vi "Output Powers Saving.vi"(7 "connection information":path, 8 "EFCVoltage":string, 9 "OutputPower":string="40000057.37", 10 "DC_SN":string, 11 "Temperature":string) -> ()   [LabVIEW 2024]
uses:
  <vilib>/addons/database/NI_Database_API.lvlib
  <vilib>/addons/database/_DB Variant To Data/Database Variant To Data.xnode
  <vilib>/addons/database/Connection.llb/DB Tools Open Connec (Path).vi
  <vilib>/addons/database/Connection.llb/Conn Execute.vi
  <vilib>/addons/database/Recordset.llb/Rec Destroy - Connection.vi
panel:
  out "Time Measured":string
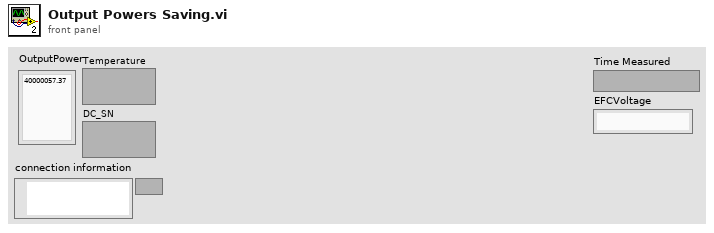
[diagram p1: front panel]
types:
  T1 = typedef "NI_Database_API.lvlib/Conn ObjectReference.ctl" = refnum<k1>
  T2 = typedef "NI_Database_API.lvlib/Rec ObjectReference.ctl" = refnum<k1>
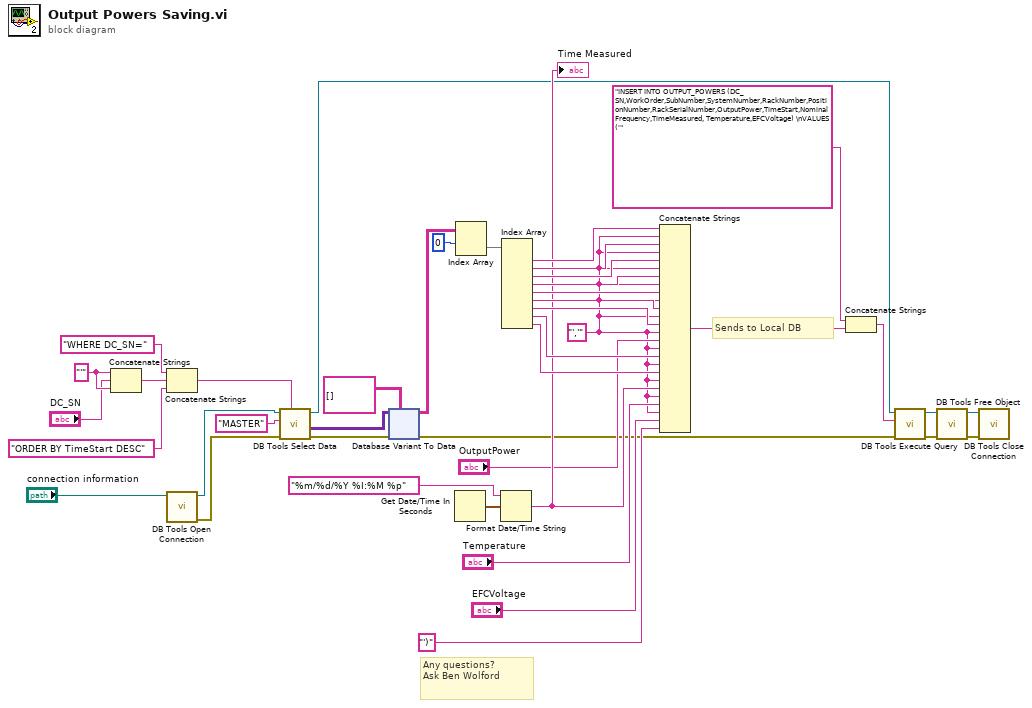
[diagram p0: block diagram]
diagram:
  w23 = "'" ("string")
  w18 = "','"
  # "Sends to Local DB"
  # "Any questions? \nAsk Ben Wolford"
  n1 = Concatenate Strings(w23, "DC_SN", w23) -> (w21:string)
  n2 = Concatenate Strings("WHERE DC_SN=" ("SQL Query"), w21, "ORDER BY TimeStart DESC" ("string")) -> (w9:string)
  n3 = call-poly <vilib>:"DB Tools Open Connection.vi"("connection information"="connection information") -> ("error out"=w15:errorcluster, "connection reference"=w16:T1)  [unwired: 7 in]
  n4 = call <vilib>:"DB Tools Select Data.vi"("condition"=w9, "error in (no error)"=w15, "table"="MASTER", "connection reference"=w16) -> ("error out"=w14:errorcluster, "data"=w12:variant[][], "connection reference out"=w6:T1)  [unwired: 2 in]
  n5 = xnode "Database Variant To Data"("database variant"=w12, "error in (no error)"=w14, "type"=string[][] [] ("DC.SN")) -> ("data"=w8:string[][], "error out"=w7:errorcluster)
  n6 = Get Date/Time In Seconds() -> (seconds since 1Jan1904=w38:timestamp)
  n7 = Index Array(array=w8, index (row)=0 ("disabled index (row)")) -> (element=w40:string[])  [unwired: 1 in]
  n8 = Format Date/Time String(time format string (%c)="%m/%d/%Y %I:%M %p", seconds (now)=w38) -> (date/time string=w24:string)  [unwired: 1 in]
  "Time Measured" <- w24
  n9 = Index Array(array=w40) -> (element #1=w36:string, element #2=w35:string, element #3=w34:string, element #4=w33:string, element #5=w26:string, element #6=w25:string, element #7=w30:string, element #8=w42:string, element #9=w27:string)  [unwired: 9 in]
  n10 = Concatenate Strings(w36, w18, w35, w18, w34, w18, w33, w18, w26, w18, w25, w18, w30, w18, "OutputPower", w18, w42, w18, w27, w18, w24, w18, "Temperature", w18, "EFCVoltage", "')" ("string")) -> (w39:string)
  n11 = Concatenate Strings("INSERT INTO OUTPUT_POWERS (DC_SN,WorkOrder,SubNumber,SystemNumber,RackNumber,PositionNumber,RackSerialNumber,OutputPower,TimeStart,NominalFrequency,TimeMeasured, Temperature,EFCVoltage) \nVALUES ('" ("string"), w39) -> (w1:string)
  n12 = call-poly <vilib>:"DB Tools Execute Query.vi"("error in (no error)"=w7, "SQL query"=w1, "connection reference"=w6) -> ("error out"=w4:errorcluster, "recordset reference"=w5:T2)  [unwired: 5 in]
  n13 = call-poly <vilib>:"DB Tools Free Object.vi"("error in (no error)"=w4, "recordset reference"=w5) -> ("error out"=w2:errorcluster, "connection reference"=w3:T1)  [unwired: 8 in]
  n14 = call <vilib>:"DB Tools Close Connection.vi"("error in (no error)"=w2, "connection reference"=w3) -> ()  [unwired: 5 in, 1 out]
